vi "Registers.vi"(0 "register instruction":T6, 5 "config.resources":T4, 7 "sync.resources":T7, 9 "time.resources":T3) -> (4 "read completion out":T5, 14 "ready for input":bool)   [LabVIEW 2021]
doc: "Sets/gets the configuration values for the instrument design libraries by connecting them to the Register Bus.\n\n<B>Input Parameters</B>\n\n<B>register instruction</B> is the register bus instruction to execute.\n\n<B>config.resources</B> are references to the configuration registers.\n\n<B>sync.resources</B> are references to the synchronization registers.\n\n<B>time.resources</B> are references to the time registers.\n\n<B>Output Parameters</B>\n\n<B>read completion out</B> is the output of the last executed register instruction.\n\n<B>ready for input</B> is a flow control signal that indicates whether the Registers VI is ready to accept a new instruction."
uses:
  <instrlib>/niUsrpRio/Synchronization/v1/FPGA/Private/Resources.ctl
  <instrlib>/_niInstr/Register Bus/v1/FPGA/Public/Register Instruction.ctl
  <instrlib>/_niInstr/Register Bus/v1/FPGA/Public/Read Completion.ctl
  <instrlib>/niUsrpRio/Time/v1/FPGA/Private/Time Resources.ctl
  <instrlib>/niUsrpRio/Time/v1/FPGA/Private/Future Event Resources.ctl
  <instrlib>/_niInstr/Register Bus/v1/FPGA/Private/Mux/Read Completion Mux (8 inputs).vi
  <instrlib>/_niInstr/Register Bus/v1/FPGA/niInstr Register Bus v1 FPGA.lvlib
  <instrlib>/niUsrpRio/GPS/v1/FPGA/niUsrpRio GPS v1 FPGA.lvlib
  <instrlib>/niUsrpRio/Config/v1/FPGA/niUsrpRio Config v1 FPGA.lvlib
  <instrlib>/niUsrpRio/Time/v1/FPGA/niUsrpRio Time v1 FPGA.lvlib
  <instrlib>/niUsrpRio/Synchronization/v1/FPGA/niUsrpRio Synchronization v1 FPGA.lvlib
  <instrlib>/niUsrpRio/Instruction Synchronizer/v1/FPGA/niUsrpRio Instruction Synchronizer v1 FPGA.lvlib
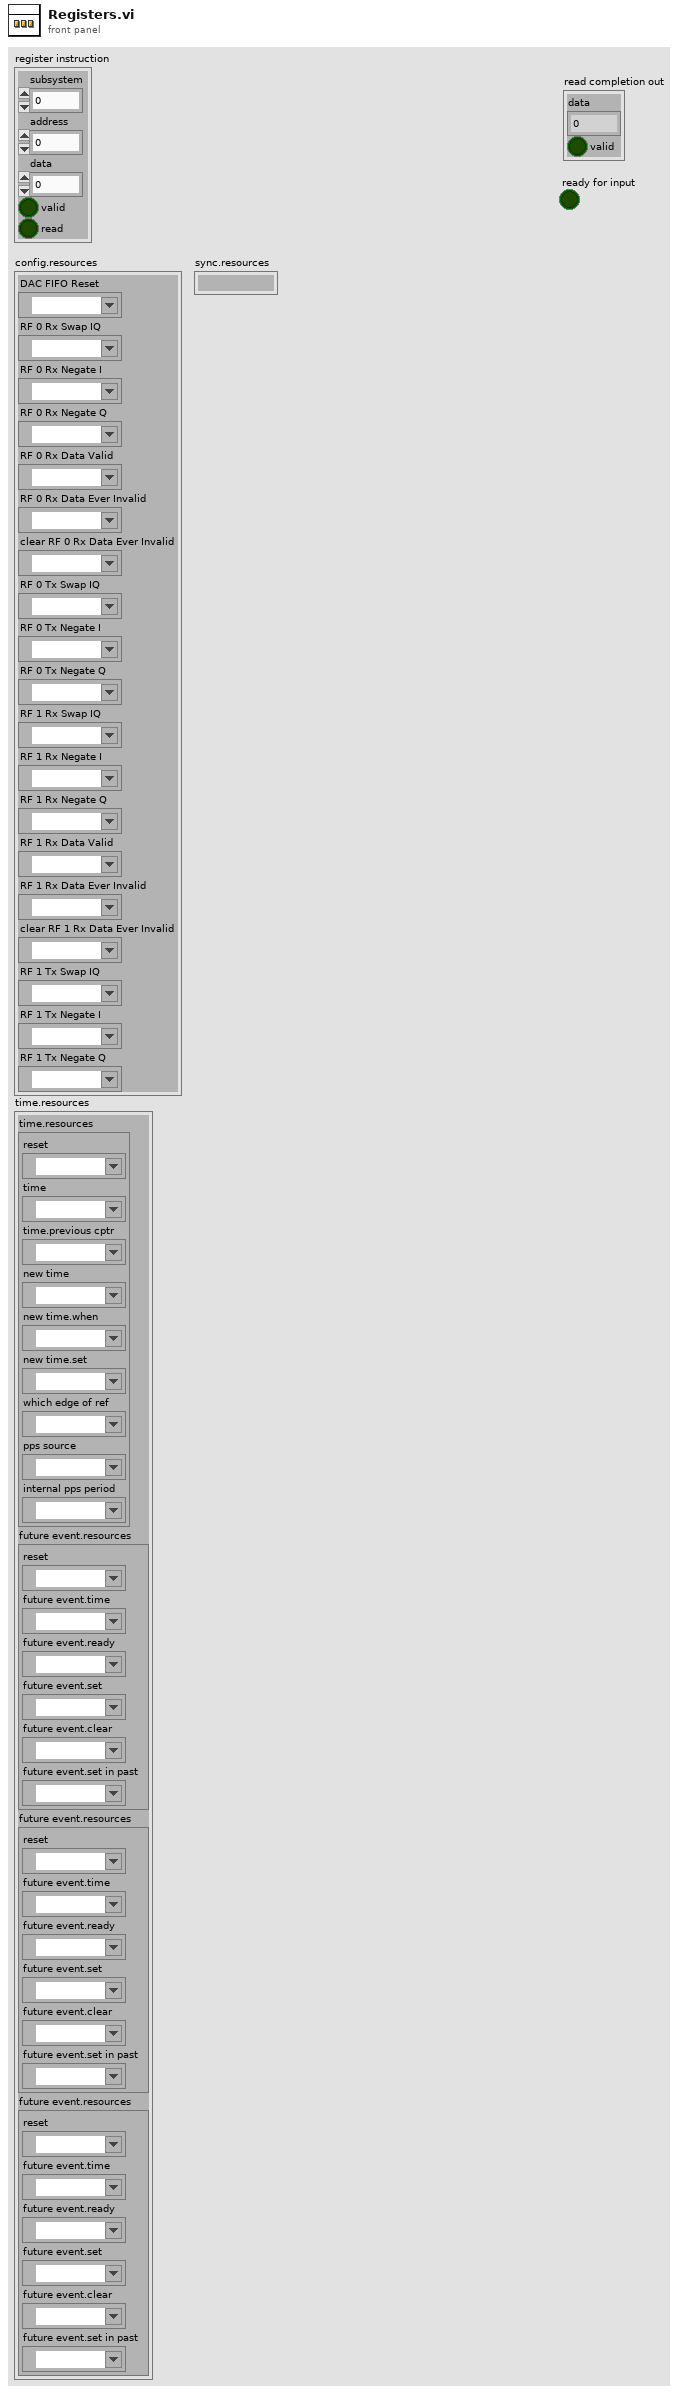
[diagram p1: front panel]
types:
  T1 = typedef "niUsrpRio Time v1 FPGA.lvlib/Time Resources.ctl" = cluster{"reset":refnum<k21>, "time":refnum<k21>, "time.previous cptr":refnum<k21>, "new time":refnum<k21>, "new time.when":refnum<k21>, "new time.set":refnum<k21>, "which edge of ref":refnum<k21>, "pps source":refnum<k21>, "internal pps period":refnum<k21>}
  T2 = typedef "niUsrpRio Time v1 FPGA.lvlib/Future Event Resources.ctl" = cluster{"reset":refnum<k21>, "future event.time":refnum<k21>, "future event.ready":refnum<k21>, "future event.set":refnum<k21>, "future event.clear":refnum<k21>, "future event.set in past":refnum<k21>}
  T3 = cluster{"time.resources":T1, "future event.resources":T2, "future event.resources":T2, "future event.resources":T2}
  T4 = cluster{"DAC FIFO Reset":refnum<k21>, "RF 0 Rx Swap IQ":refnum<k21>, "RF 0 Rx Negate I":refnum<k21>, "RF 0 Rx Negate Q":refnum<k21>, "RF 0 Rx Data Valid":refnum<k21>, "RF 0 Rx Data Ever Invalid":refnum<k21>, "clear RF 0 Rx Data Ever Invalid":refnum<k21>, "RF 0 Tx Swap IQ":refnum<k21>, "RF 0 Tx Negate I":refnum<k21>, "RF 0 Tx Negate Q":refnum<k21>, "RF 1 Rx Swap IQ":refnum<k21>, "RF 1 Rx Negate I":refnum<k21>, "RF 1 Rx Negate Q":refnum<k21>, "RF 1 Rx Data Valid":refnum<k21>, "RF 1 Rx Data Ever Invalid":refnum<k21>, "clear RF 1 Rx Data Ever Invalid":refnum<k21>, "RF 1 Tx Swap IQ":refnum<k21>, "RF 1 Tx Negate I":refnum<k21>, "RF 1 Tx Negate Q":refnum<k21>}
  T5 = typedef "niInstr Register Bus v1 FPGA.lvlib/Read Completion.ctl" = cluster{"data":u32, "valid":bool}
  T6 = typedef "niInstr Register Bus v1 FPGA.lvlib/Register Instruction.ctl" = cluster{"subsystem":u8, "address":u16, "data":u32, "valid":bool, "read":bool}
  T7 = typedef "niUsrpRio Synchronization v1 FPGA.lvlib/Resources.ctl" = cluster{"master":refnum<k21>, "meas.enable":refnum<k21>, "meas.ready":refnum<k21>, "meas.reset":refnum<k21>, "meas.arm":refnum<k21>, "meas.valid":refnum<k21>, "meas.value":refnum<k21>, "meas.oversample factor":refnum<k21>, "cptr":refnum<k21>, "cptr.adjust":refnum<k21>, "cptr.period":refnum<k21>}
  T8 = enum8{"rx.start trigger event", "tx.start trigger event", "instruction synchronizer event"}
  T9 = cluster{"read completion":T5, "read completion":T5, "read completion":T5, "read completion":T5}
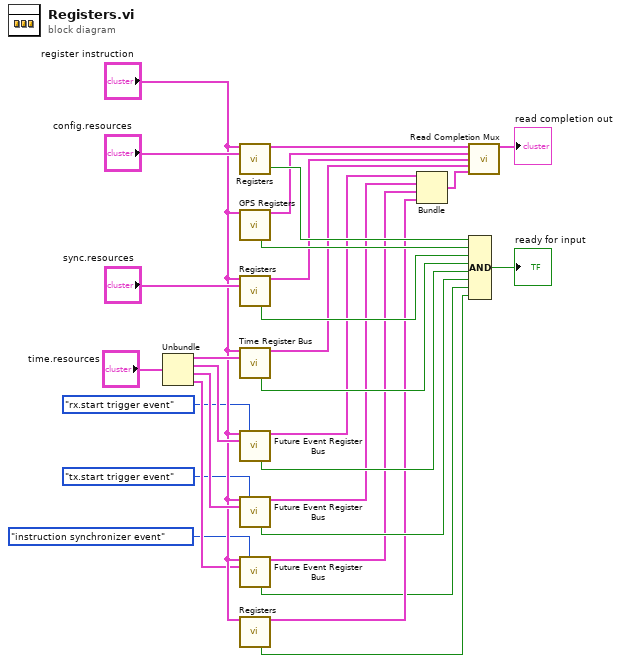
[diagram p0: block diagram]
diagram:
  n1 = Unbundle("time.resources") -> ("time.resources"=w14:T1, "future event.resources"=w13:T2, "future event.resources"=w12:T2, "future event.resources"=w8:T2)
  n2 = call <instrlib>:"Registers.vi"("register instruction"="register instruction", "resources"="config.resources") -> ("read completion out"=w18:T5, "ready for input"=w25:bool)  [unwired: 12 in]
  n3 = call <instrlib>:"GPS Registers.vi"("register instruction"="register instruction") -> ("read completion"=w19:T5, "ready for input"=w26:bool)  [unwired: 13 in]
  n4 = call <instrlib>:"Registers.vi"("register instruction"="register instruction", "sync.resources"="sync.resources") -> ("read completion"=w23:T5, "ready for input"=w27:bool)  [unwired: 12 in]
  n5 = call <instrlib>:"Time Register Bus.vi"("register instruction"="register instruction", "time.resources"=w14) -> ("read completion"=w22:T5, "ready for input"=w28:bool)  [unwired: 12 in]
  n6 = call <instrlib>:"Future Event Register Bus.vi"("register instruction"="register instruction", "instance"=T8."rx.start trigger event", "future event.resources"=w13) -> ("read completion"=w20:T5, "ready for input"=w29:bool)  [unwired: 11 in]
  n7 = call <instrlib>:"Future Event Register Bus.vi"("register instruction"="register instruction", "instance"=T8."tx.start trigger event", "future event.resources"=w12) -> ("read completion"=w11:T5, "ready for input"=w30:bool)  [unwired: 11 in]
  n8 = call <instrlib>:"Future Event Register Bus.vi"("register instruction"="register instruction", "instance"=T8."instruction synchronizer event", "future event.resources"=w8) -> ("read completion"=w7:T5, "ready for input"=w5:bool)  [unwired: 11 in]
  n9 = call <instrlib>:"Registers.vi"("register instruction"="register instruction") -> ("read completion"=w6:T5, "ready for input"=w4:bool)  [unwired: 13 in]
  n10 = Bundle("read completion"=w20, "read completion"=w11, "read completion"=w7, "read completion"=w6) -> (w21:T9)  [unwired: 1 in]
  n11 = call-poly <instrlib>:"Read Completion Mux.vi"("element 0"=w18, "element 1"=w19, "element 2"=w23, "element 3"=w22, "remaining elements (cluster)"=w21) -> ("read completion out"=→"read completion out":T5)  [unwired: 10 in]
  n12 = Compound Arithmetic op=AND(w25, w26, w27, w28, w29, w30, w5, w4) -> (→"ready for input":bool)
